vi "4.vi"() -> ()   [LabVIEW 2013]
uses:
  <vilib>/picture/cartesn2.llb/XY Plot Type.ctl
panel:
  out "2D Picture":picture
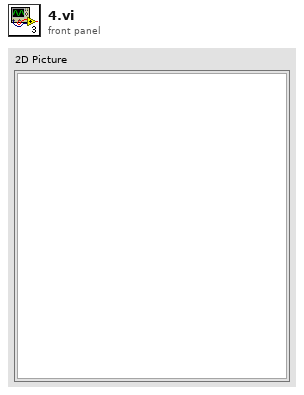
[diagram p1: front panel]
types:
  T1 = typedef "XY Plot Type.ctl" = enum16{"points", "squares", "circles", "connected points", "connected squares", "connected circles", "comb plot", "sized scatter plot", "sized-colored scatter plot", "min-max lines"}
  T2 = cluster{"plot color":u32, "XY plot type":T1, "baseline":dbl}[]
  T3 = typedef "LVBoundsTypeDef.ctl" = cluster{"Width":u32, "Height":u32}
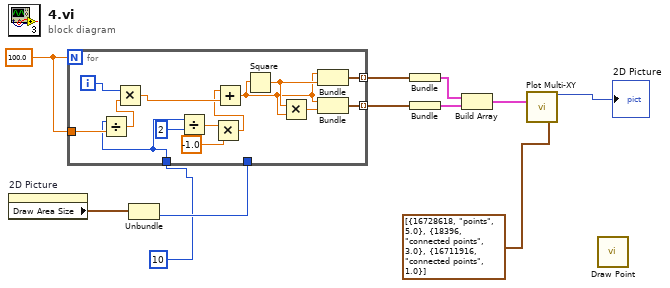
[diagram p0: block diagram]
diagram:
  w3 = 100.0
  n1 = property on="2D Picture" class="Pict"() -> ("Draw Area Size"=w4:T3)  [unwired: 2 in, 2 out]
  n2 = Unbundle(w4) -> ("Height"=w2:u32)  [unwired: 1 out]
  n3 = for {
    N: w3 -> [_]
    tunnel: [w25] -> w10 mode=indexing
    tunnel: [w21] -> w7 mode=indexing
    tunnel: u32 10 ("Width") -> [w16]
    tunnel: w3 -> [w19]
    tunnel: w2 -> [_]
    i -> [w20]
    n4 = Divide(x=w16, y=w19) -> (x/y=w18:dbl)
    n5 = Multiply(x=w20, y=w18) -> (x*y=w17:dbl)
    n6 = Divide(x=w16, y=u32 2) -> (x/y=w14:dbl)
    n7 = Multiply(x=w14, y=-1.0) -> (x*y=w12:dbl)
    n8 = Add(x=w12, y=w17) -> (x+y=w23:dbl)
    n9 = Square(x=w23) -> (x^2=w24:dbl)
    n10 = Multiply(x=w24, y=w23) -> (x*y=w22:dbl)
    n11 = Bundle(w23, w24) -> (w25:cluster{dbl, dbl})  [unwired: 1 in]
    n12 = Bundle(w23, w22) -> (w21:cluster{dbl, dbl})  [unwired: 1 in]
  }
  n13 = Bundle(w10) -> (w9:cluster{cluster{dbl, dbl}[]})  [unwired: 1 in]
  n14 = Bundle(w7) -> (w6:cluster{cluster{dbl, dbl}[]})  [unwired: 1 in]
  n15 = Build Array(w9, w6) -> (w8:cluster{cluster{dbl, dbl}[]}[])
  n16 = call <vilib>:"Plot Multi-XY.vi"("data"=w8, "XY plot cosmetics"=T2 [{"plot color"=16728618, "XY plot type"=enum."points", "baseline"=5.0}, {"plot color"=18396, "XY plot type"=enum."connected points", "baseline"=3.0}, {"plot color"=16711916, "XY plot type"=enum."connected points", "baseline"=1.0}]) -> ("new picture"=→"2D Picture":picture)  [unwired: 13 in]
  n17 = call <vilib>:"Draw Point.vi"() -> ()  [unwired: 9 in, 1 out]
